vi "moveM1motor.vi"() -> ()   [LabVIEW 2017]
uses:
  C:/GitHub/Sandbox/deltamovectrl/deltamovectrl/bin/Debug/netstandard1.4/deltamovectrl.dll
  deltamovectrl/deltamovectrl/bin/Debug/netstandard1.4/deltamovectrl.dll
panel:
  out "Boolean":bool
  in  "Speed":dbl(knob) scale=0.0..3.0
  out "?":bool
  out "?":bool
  out "Meter":dbl(knob) scale=-3.0..3.0
  in  "?":bool
  in  "?":bool
  in  "CW":bool
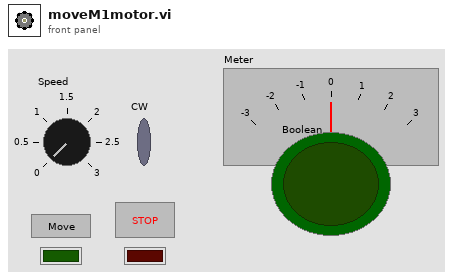
[diagram p1: front panel]
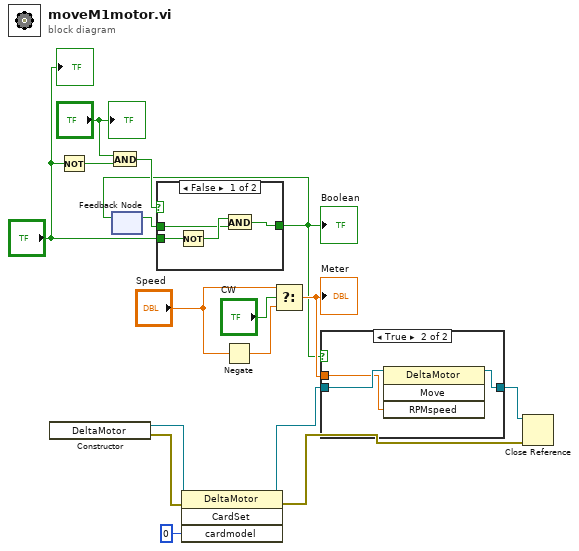
[diagram p0: block diagram]
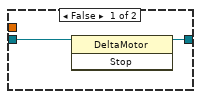
[diagram p2: hidden frame]
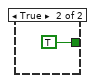
[diagram p3: hidden frame]
diagram:
  n1 = constructor class="DeltaMotor"() -> (reference out=w3:refnum<k24>, error out=w5:errorcluster)  [unwired: 3 in, 1 out]
  n2 = Not(x="?") -> (.not. x?=w13:bool)
  n3 = And(x="?", y=w13) -> (x .and. y?=w12:bool)
  n4 = feedback #1() -> (w11:bool)  [unwired: 1 in]
  n5 = case shown="False" w12 {
    tunnel: [w19 TRUE] -> w6
    tunnel: w11 -> [w18 _]
    tunnel: "?" -> [w17 _]
    frame False {
      n6 = Not(x=w17) -> (.not. x?=w20:bool)
      n7 = And(x=w20, y=w18) -> (x .and. y?=w19:bool)
    }
    frame True {
    }
  }
  "Boolean" <- w6
  n8 = feedback-in #1(w6) -> ()
  n9 = invoke class="DeltaMotor" method="CardSet"(reference=w3, error in=w5, "cardmodel"=0) -> (reference out=w2:refnum<k24>, error out=w4:errorcluster)  [unwired: 1 in, 2 out]
  n10 = Negate(x="Speed") -> (-x=w16:dbl)
  n11 = Select(t="Speed", s="CW", f=w16) -> (s? t:f=w10:dbl)
  "Meter" <- w10
  n12 = case shown="True" w6 {
    tunnel: w2 -> [w23 w26]
    tunnel: w10 -> [_ w25]
    tunnel: [w22 w24] -> w14
    frame False {
      n13 = invoke class="DeltaMotor" method="Stop"(reference=w23) -> (reference out=w22:refnum<k24>)  [unwired: 2 in, 2 out]
    }
    frame True {
      n14 = invoke on="Invoke Node" class="DeltaMotor" method="Move"(reference=w26, "RPMspeed"=w25) -> (reference out=w24:refnum<k24>)  [unwired: 2 in, 3 out]
    }
  }
  n15 = Close Reference(reference=w14, error in (no error)=w4) -> ()  [unwired: 1 out]
  "?" <- "?"
  "?" <- "?"
